vi "ArrayNotesMarcoGonzalez.vi"() -> ()   [LabVIEW 2012]
panel:
  out "Element i":dbl
  in  "stop":bool
  out "Array 2":dbl[](array[numeric])
  out "Column j":dbl
  out "Row i":dbl
  out "Array":dbl[][](array[numeric])
  # "Marco Gonzalez\nEA 3 \n03 / 09 / 2017"
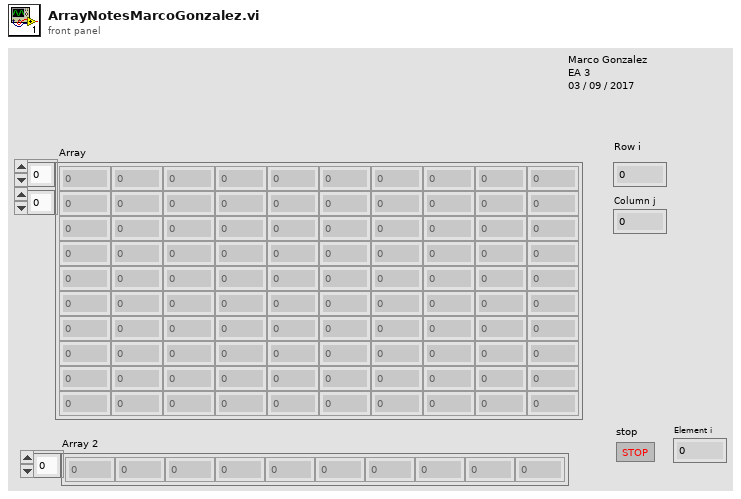
[diagram p1: front panel]
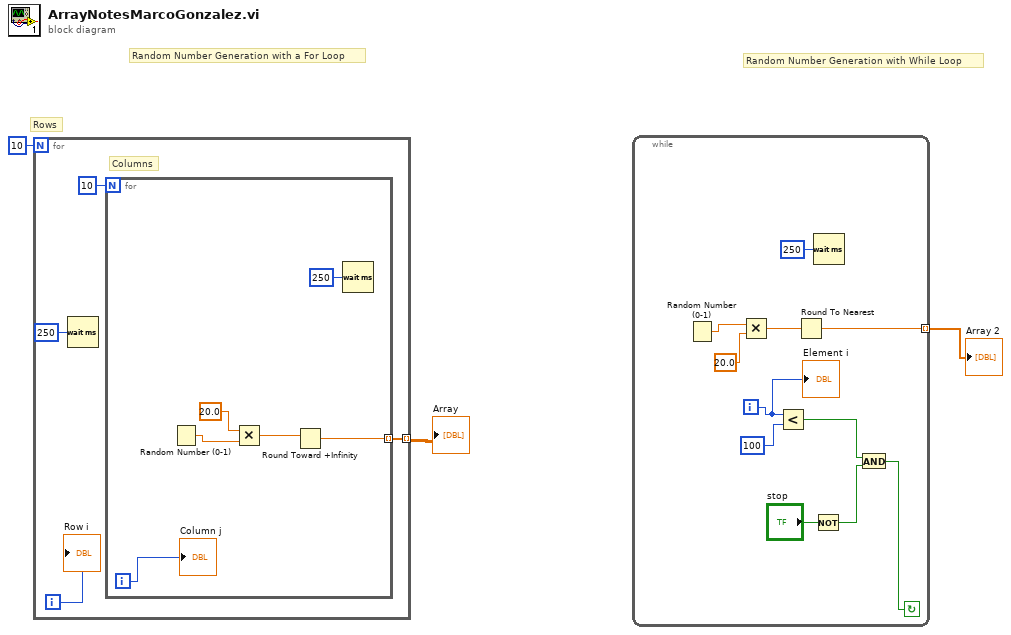
[diagram p0: block diagram]
diagram:
  # "Random Number Generation with While Loop"
  # "Random Number Generation with a For Loop"
  # "Rows"
  n1 = for {
    N: 10 -> [_]
    tunnel: [w6] -> w2 mode=indexing
    i -> [w5]
    # "Columns"
    n2 = Wait (ms)(milliseconds to wait=u32 250) -> ()  [unwired: 1 out]
    n3 = for {
      N: 10 -> [_]
      tunnel: [w10] -> w6 mode=indexing
      i -> [w9]
      n4 = Random Number (0-1)() -> (number: 0 to 1=w13:dbl)
      n5 = Multiply(x=20.0, y=w13) -> (x*y=w11:dbl)
      n6 = Round Toward +Infinity(x=w11) -> (ceil(x): smallest int >= x=w10:dbl)
      n7 = Wait (ms)(milliseconds to wait=u32 250) -> ()  [unwired: 1 out]
      "Column j" <- w9
    }
    "Row i" <- w5
  }
  "Array" <- w2
  n8 = while {
    tunnel: [w21] -> w1 mode=indexing
    i -> [w15]
    stop <- w16 continue-if-true
    n9 = Random Number (0-1)() -> (number: 0 to 1=w23:dbl)
    n10 = Multiply(x=w23, y=20.0) -> (x*y=w22:dbl)
    n11 = Less?(x=w15, y=100) -> (x < y?=w17:bool)
    n12 = Round To Nearest(number=w22) -> (nearest integer value=w21:dbl)
    n13 = Not(x="stop") -> (.not. x?=w18:bool)
    n14 = Wait (ms)(milliseconds to wait=u32 250) -> ()  [unwired: 1 out]
    n15 = And(x=w17, y=w18) -> (x .and. y?=w16:bool)
    "Element i" <- w15
  }
  "Array 2" <- w1
